vi "PIDmaker.vi"(0 "New Time":sgl, 1 "Kp":sgl, 2 "Kd":sgl, 3 "Ki":sgl, 5 "Old Time":sgl, 7 "New Value":sgl, 9 "Old Value":sgl, 11 "Desired Value":sgl, 12 "Integral In":sgl) -> (4 "P out":sgl, 6 "D out":sgl, 8 "I out":sgl, 14 "Integral Out":sgl)   [LabVIEW 2016]
doc: "Consolidates Integral and Derivative Calculations, Error Calculations, and Component Summing into a single block. \n\nOld Value/Time must be updated from a shift register output, which takes New Value/Time as an input.\n\nIntegral Out must be connected to Integral In via a shift register."
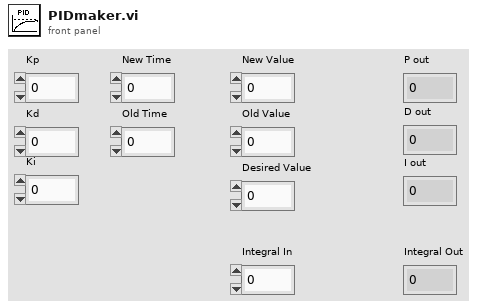
[diagram p1: front panel]
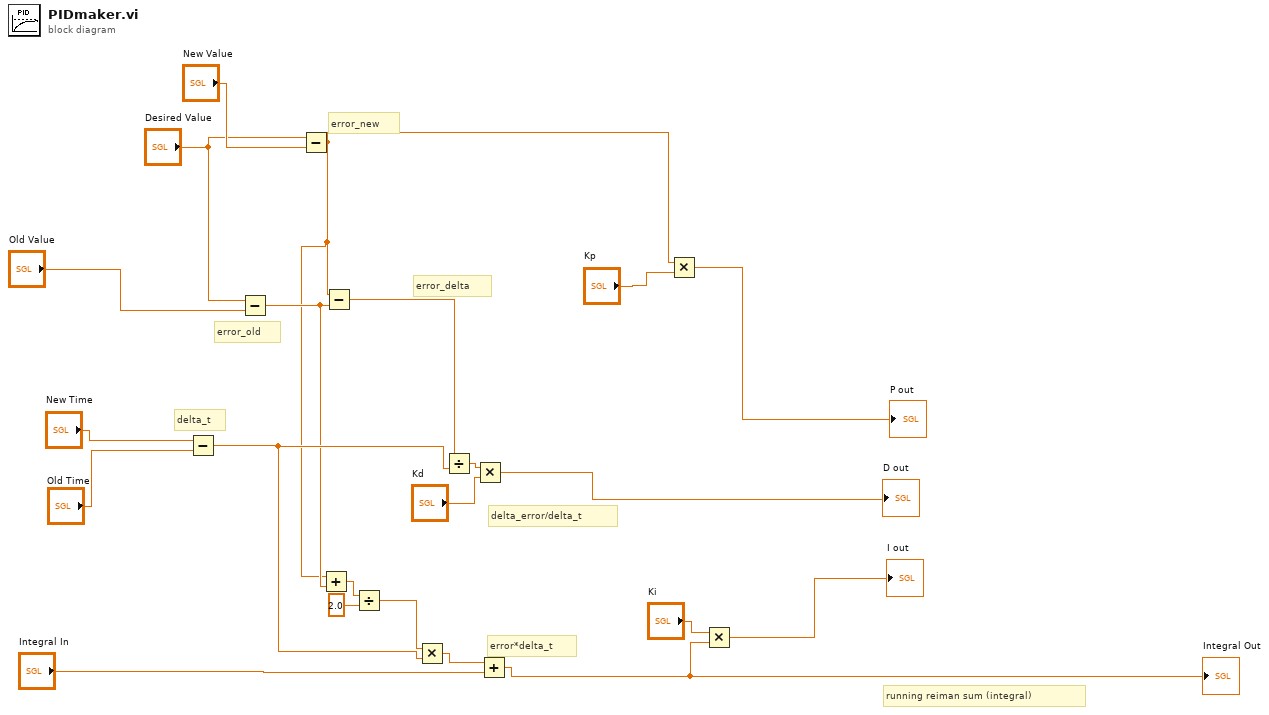
[diagram p0: block diagram]
diagram:
  # "error*delta_t"
  # "delta_error/delta_t"
  # "running reiman sum (integral)"
  # "error_delta"
  # "error_old"
  # "error_new"
  # "delta_t"
  n1 = Subtract(x="New Time", y="Old Time") -> (x-y=w6:sgl)
  n2 = Subtract(x="Desired Value", y="Old Value") -> (x-y=w5:sgl)
  n3 = Subtract(x="Desired Value", y="New Value") -> (x-y=w4:sgl)
  n4 = Add(x=w4, y=w5) -> (x+y=w3:sgl)
  n5 = Subtract(x=w4, y=w5) -> (x-y=w16:sgl)
  n6 = Divide(x=w3, y=sgl 2.0) -> (x/y=w1:sgl)
  n7 = Multiply(x=w1, y=w6) -> (x*y=w19:sgl)
  n8 = Divide(x=w16, y=w6) -> (x/y=w15:sgl)
  n9 = Multiply(x=w15, y="Kd") -> (x*y=→"D out":sgl)
  n10 = Add(x=w19, y="Integral In") -> (x+y=w11:sgl)
  "Integral Out" <- w11
  n11 = Multiply(x=w4, y="Kp") -> (x*y=→"P out":sgl)
  n12 = Multiply(x="Ki", y=w11) -> (x*y=→"I out":sgl)
